vi "Output Waveforms.vi"(4 "Transition Active?":bool, 5 "Mode":string, 6 "Setpoint":dbl, 7 "Simulated Sensor Injection":dbl, 8 "error in (no error)":errorcluster, 9 "Previous Setpoint":dbl, 10 "Instrument Specifications":T2, 11 "Refnum in":refnum<k21>) -> (0 "error out":errorcluster, 1 "data":waveform(dbl)[](array[waveform]), 2 "UUT Display Data":T1, 3 "Refnum out":refnum<k21>)   [LabVIEW 2026, in "Acquisition.lvlib"]
uses:
  Acquisition.lvlib
  Instrument Specifications Configuration.ctl
  Instrument Specifications Cluster Configuration.ctl
  controls/UI/Measurement Role.ctl
  controls/UI/UUT Display Data.ctl
  <vilib>/DAQmx/read.llb/DAQmx Read (Analog 1D Wfm NChan NSamp).vi
  <vilib>/DAQmx/miscellaneous.llb/DAQmx Fill In Error Info.vi
  Settings/Settings.lvlib
  <vilib>/Analysis/NI_AALBase.lvlib
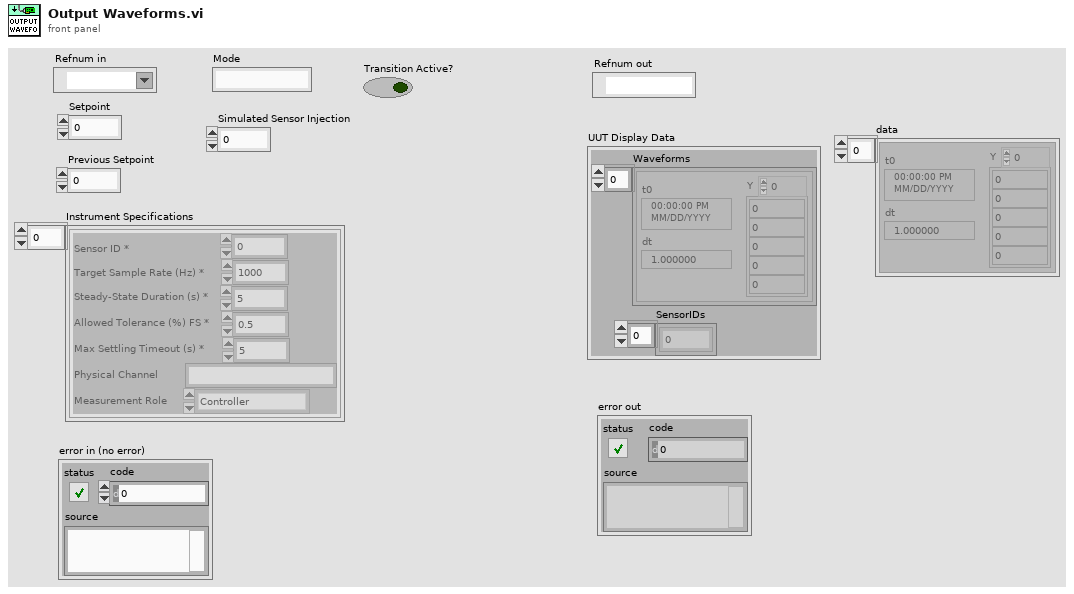
[diagram p1: front panel]
types:
  T1 = typedef "UUT Display Data.ctl" = cluster{"Waveforms":waveform(dbl)[], "SensorIDs":i32[]}
  T2 = typedef "Acquisition.lvlib/Instrument Specifications Configuration.ctl" = T3[]
  T3 = typedef "Acquisition.lvlib/Instrument Specifications Cluster Configuration.ctl" = cluster{"Sensor ID *":i32, "Target Sample Rate (Hz) *":dbl, "Steady-State Duration (s) *":i32, "Allowed Tolerance (%) FS *":dbl, "Max Settling Timeout (s) *":i32, "Physical Channel":string, "Measurement Role":T4}
  T4 = typedef "Settings.lvlib/Measurement Role.ctl" = enum16{"Controller", "Reference", "UUT"}
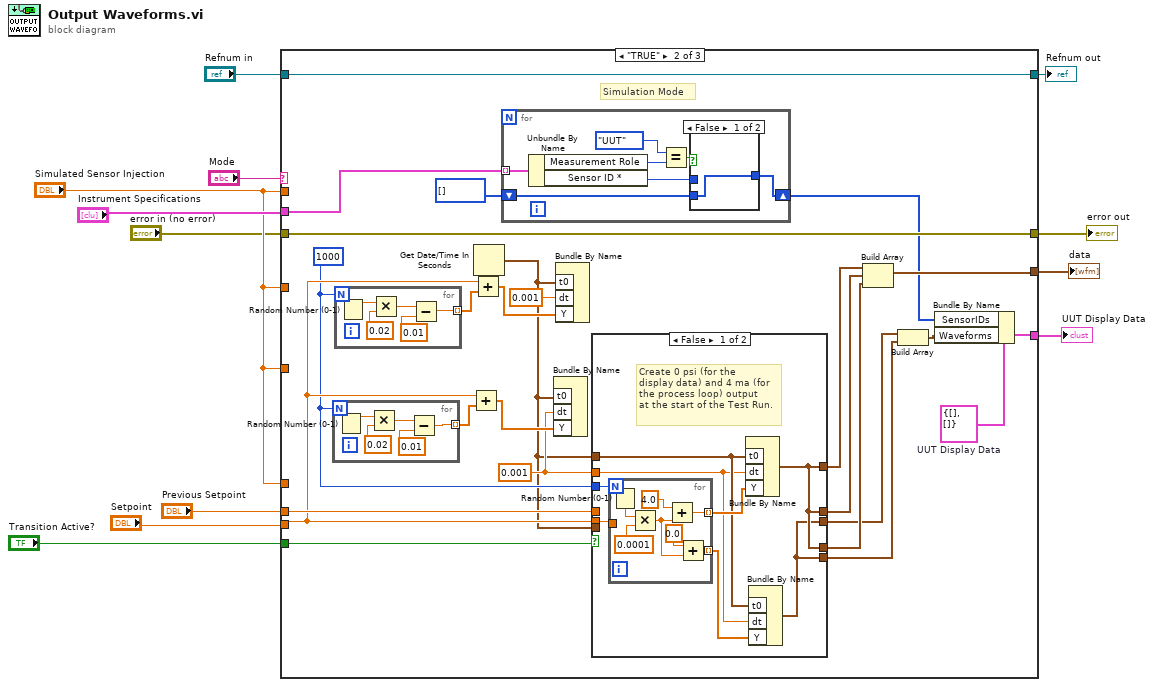
[diagram p0: block diagram]
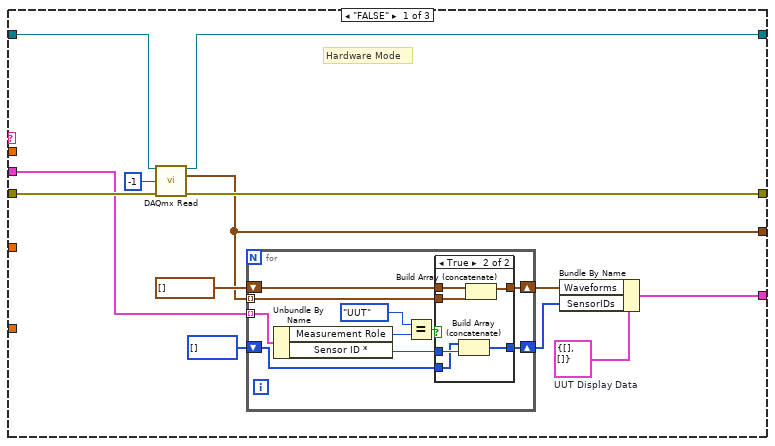
[diagram p2: hidden frame]
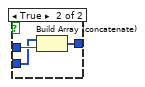
[diagram p4: hidden frame]
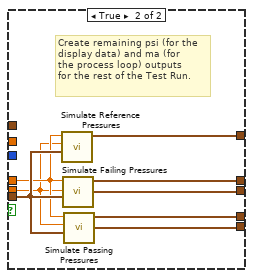
[diagram p5: hidden frame]
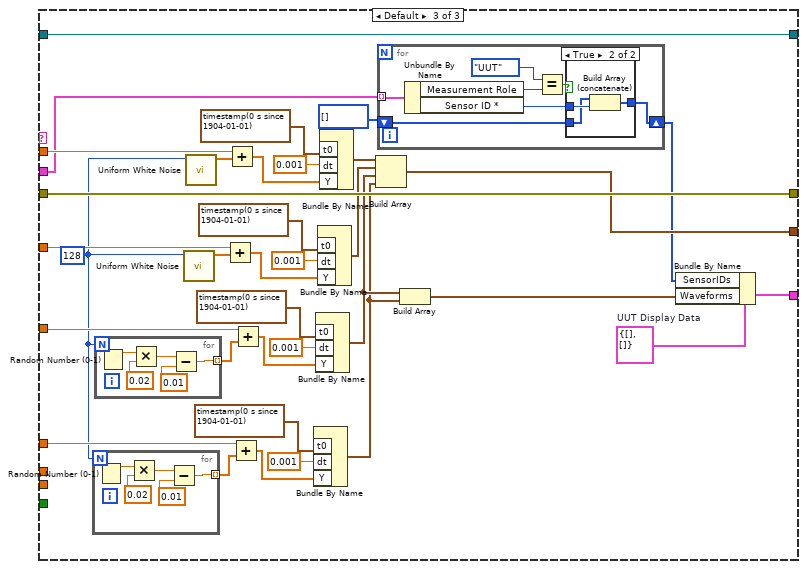
[diagram p6: hidden frame]
diagram:
  n1 = case shown="\"TRUE\"" "Mode" {
    tunnel: "Refnum in" -> [w25 w68 w145]
    tunnel: [w22 w68 w145] -> w3
    tunnel: "error in (no error)" -> [w23 w62 w143]
    tunnel: [w21 w62 w143] -> w10
    tunnel: [w13 w47 w114] -> w5
    tunnel: "Simulated Sensor Injection" -> [_ _ w142]
    tunnel: "Simulated Sensor Injection" -> [_ _ w134]
    tunnel: "Simulated Sensor Injection" -> [_ _ w131]
    tunnel: "Simulated Sensor Injection" -> [_ _ w122]
    tunnel: "Previous Setpoint" -> [_ w61 _]
    tunnel: "Setpoint" -> [_ w60 _]
    tunnel: "Transition Active?" -> [_ w59 _]
    tunnel: "Instrument Specifications" -> [w20 w52 w117]
    tunnel: [w18 w53 w118] -> w12
    frame "FALSE" {
      w16 = T1 {"Waveforms"=[], "SensorIDs"=[]}  # UUT Display Data
      # "Hardware Mode"
      n2 = call-poly <vilib>:"DAQmx Read.vi"("task/channels in"=w25, "number of samples per channel"=-1, "error in"=w23) -> ("task out"=w22:refnum<k21>, "data"=w18:waveform(dbl)[], "error out"=w21:errorcluster)  [unwired: 10 in]
      n3 = for {
        tunnel: w20 -> [w35] mode=indexing
        tunnel: w18 -> [w33] mode=indexing
        shift-right: [w32] -> w15
        shift-left: waveform(dbl)[] [] -> [w31]
        shift-right: [w27] -> w14
        shift-left: i32[] [] -> [w26]
        n4 = Unbundle By Name(w35) -> ("Measurement Role"=w29:T4, "Sensor ID *"=w28:i32)
        n5 = Equal?(x=Measurement_Role."UUT" ("Measurement Role"), y=w29) -> (x = y?=w34:bool)
        n6 = case shown="True" w34 {
          tunnel: w33 -> [_ w43]
          tunnel: [w37 w42] -> w32
          tunnel: w31 -> [w37 w41]
          tunnel: w28 -> [_ w40]
          tunnel: [w36 w39] -> w27
          tunnel: w26 -> [w36 w38]
          frame False {
          }
          frame True {
            n7 = Build Array (concatenate)(w38, w40) -> (w39:i32[])
            n8 = Build Array (concatenate)(w41, w43) -> (w42:waveform(dbl)[])
          }
        }
      }
      n9 = Bundle By Name(cluster=w16, "Waveforms"=w15, "SensorIDs"=w14) -> (w13:T1)
    }
    frame "TRUE" {
      w50 = T1 {"Waveforms"=[], "SensorIDs"=[]}  # UUT Display Data
      w58 = 1000
      w57 = 0.001 ("dt")
      # "Simulation Mode"
      n10 = for {
        N: w58 -> [_]
        tunnel: [w103] -> w63 mode=indexing
        n11 = Random Number (0-1)() -> (number: 0 to 1=w106:dbl)
        n12 = Multiply(x=w106, y=0.02) -> (x*y=w105:dbl)
        n13 = Subtract(x=w105, y=0.01) -> (x-y=w103:dbl)
      }
      n14 = for {
        N: w58 -> [_]
        tunnel: [w108] -> w65 mode=indexing
        n15 = Random Number (0-1)() -> (number: 0 to 1=w111:dbl)
        n16 = Multiply(x=w111, y=0.02) -> (x*y=w110:dbl)
        n17 = Subtract(x=w110, y=0.01) -> (x-y=w108:dbl)
      }
      n18 = Add(x=w60, y=w63) -> (x+y=w64:dbl[])
      n19 = Add(x=w60, y=w65) -> (x+y=w66:dbl[])
      n20 = Get Date/Time In Seconds() -> (seconds since 1Jan1904=w56:timestamp)
      n21 = for {
        tunnel: w52 -> [w75] mode=indexing
        shift-right: [w70] -> w49
        shift-left: i32[] [] -> [w69]
        n22 = Unbundle By Name(w75) -> ("Measurement Role"=w72:T4, "Sensor ID *"=w71:i32)
        n23 = Equal?(x=Measurement_Role."UUT" ("Measurement Role"), y=w72) -> (x = y?=w74:bool)
        n24 = case shown="False" w74 {
          tunnel: w71 -> [_ w79]
          tunnel: [w76 w78] -> w70
          tunnel: w69 -> [w76 w77]
          frame False {
          }
          frame True {
            n25 = Build Array (concatenate)(w77, w79) -> (w78:i32[])
          }
        }
      }
      n26 = Bundle By Name("t0"=w56, "dt"=w57, "Y"=w64) -> ()  [unwired: 1 in, 1 out]
      n27 = Bundle By Name("t0"=w56, "dt"=0.001, "Y"=w66) -> ()  [unwired: 1 in, 1 out]
      n28 = case shown="False" w59 {
        tunnel: [w85 w102] -> w55
        tunnel: [w85 w101] -> w54
        tunnel: w61 -> [_ w99]
        tunnel: w60 -> [w86 w98]
        tunnel: w58 -> [w87 _]
        tunnel: w57 -> [w82 _]
        tunnel: w56 -> [w83 _]
        tunnel: w56 -> [_ w100]
        tunnel: [w85 w97] -> w46
        tunnel: [w80 w96] -> w45
        tunnel: [w80 w95] -> w44
        frame False {
          # "Create 0 psi (for the\ndisplay data) and 4 ma (for\nthe process loop) output\nat the start of the Test Run."
          n29 = for {
            N: w87 -> [_]
            tunnel: w86 -> [_]
            tunnel: [w91] -> w84 mode=indexing
            tunnel: [w88] -> w81 mode=indexing
            n30 = Random Number (0-1)() -> (number: 0 to 1=w94:dbl)
            n31 = Multiply(x=w94, y=0.0001) -> (x*y=w89:dbl)
            n32 = Add(x=4.0, y=w89) -> (x+y=w91:dbl)
            n33 = Add(x=0.0, y=w89) -> (x+y=w88:dbl)
          }
          n34 = Bundle By Name("t0"=w83, "dt"=w82, "Y"=w84) -> (w85:waveform(dbl))  [unwired: 1 in]
          n35 = Bundle By Name("t0"=w83, "dt"=w82, "Y"=w81) -> (w80:waveform(dbl))  [unwired: 1 in]
        }
        frame True {
          # "Create remaining psi (for the\ndisplay data) and ma (for\nthe process loop) outputs\nfor the rest of the Test Run."
          n36 = call "Simulate Reference Pressures.vi"("seconds since 1Jan1904"=w100, "Pf"=w98, "Pi"=w99) -> ("Simulated Waveform"=w97:waveform(dbl))  [unwired: 7 in, 1 out]
          n37 = call "Simulate Failing Pressures.vi"("seconds since 1Jan1904"=w100, "Pf"=w98, "Pi"=w99) -> ("Simulated Waveform units"=w96:waveform(dbl), "Simulated Waveform signal"=w102:waveform(dbl))  [unwired: 6 in, 1 out]
          n38 = call "Simulate Passing Pressures.vi"("seconds since 1Jan1904"=w100, "Pf"=w98, "Pi"=w99) -> ("Simulated Waveform units"=w95:waveform(dbl), "Simulated Waveform signal"=w101:waveform(dbl))  [unwired: 6 in, 1 out]
        }
      }
      n39 = Build Array(w46, w55, w54) -> (w53:waveform(dbl)[])
      n40 = Build Array(w45, w44) -> (w48:waveform(dbl)[])
      n41 = Bundle By Name(cluster=w50, "SensorIDs"=w49, "Waveforms"=w48) -> (w47:T1)
    }
    frame Default {
      w114 = T1 {"Waveforms"=[], "SensorIDs"=[]}  # UUT Display Data
      w121 = 128 ("samples")
      n42 = for {
        N: w121 -> [_]
        tunnel: [w157] -> w123 mode=indexing
        n43 = Random Number (0-1)() -> (number: 0 to 1=w160:dbl)
        n44 = Multiply(x=w160, y=0.02) -> (x*y=w159:dbl)
        n45 = Subtract(x=w159, y=0.01) -> (x-y=w157:dbl)
      }
      n46 = for {
        N: w121 -> [_]
        tunnel: [w162] -> w129 mode=indexing
        n47 = Random Number (0-1)() -> (number: 0 to 1=w165:dbl)
        n48 = Multiply(x=w165, y=0.02) -> (x*y=w164:dbl)
        n49 = Subtract(x=w164, y=0.01) -> (x-y=w162:dbl)
      }
      n50 = call <vilib>:"Uniform White Noise.vi"("samples"=w121) -> ("uniform white noise"=w138:dbl[])  [unwired: 9 in, 1 out]
      n51 = call <vilib>:"Uniform White Noise.vi"("samples"=w121) -> ("uniform white noise"=w144:dbl[])  [unwired: 9 in, 1 out]
      n52 = Add(x=w134, y=w138) -> (x+y=w137:dbl[])
      n53 = Add(x=w142, y=w144) -> (x+y=w141:dbl[])
      n54 = Add(x=w122, y=w123) -> (x+y=w124:dbl[])
      n55 = Add(x=w131, y=w129) -> (x+y=w130:dbl[])
      n56 = Bundle By Name("t0"=timestamp(0 s since 1904-01-01), "dt"=0.001, "Y"=w124) -> (w119:waveform(dbl))  [unwired: 1 in]
      n57 = Bundle By Name("t0"=timestamp(0 s since 1904-01-01), "dt"=0.001, "Y"=w130) -> (w120:waveform(dbl))  [unwired: 1 in]
      n58 = Bundle By Name("t0"=timestamp(0 s since 1904-01-01), "dt"=0.001, "Y"=w137) -> (w128:waveform(dbl))  [unwired: 1 in]
      n59 = Bundle By Name("t0"=timestamp(0 s since 1904-01-01), "dt"=0.001, "Y"=w141) -> (w127:waveform(dbl))  [unwired: 1 in]
      n60 = Build Array(w127, w128, w120, w119) -> (w118:waveform(dbl)[])
      n61 = for {
        tunnel: w117 -> [w152] mode=indexing
        shift-right: [w147] -> w115
        shift-left: i32[] [] -> [w146]
        n62 = Unbundle By Name(w152) -> ("Measurement Role"=w149:T4, "Sensor ID *"=w148:i32)
        n63 = Equal?(x=Measurement_Role."UUT" ("Measurement Role"), y=w149) -> (x = y?=w151:bool)
        n64 = case shown="True" w151 {
          tunnel: w148 -> [_ w156]
          tunnel: [w153 w155] -> w147
          tunnel: w146 -> [w153 w154]
          frame False {
          }
          frame True {
            n65 = Build Array (concatenate)(w154, w156) -> (w155:i32[])
          }
        }
      }
      n66 = Build Array(w120, w119) -> (w116:waveform(dbl)[])
      n67 = Bundle By Name(cluster=w114, "SensorIDs"=w115, "Waveforms"=w116) -> ()  [unwired: 1 out]
    }
  }
  "data" <- w12
  "error out" <- w10
  "UUT Display Data" <- w5
  "Refnum out" <- w3
